vi "oa_Multichannel dr Check.vi"(8 "error in (no error)":errorcluster, 11 "resampled signal in":cluster{"r0":dbl, "dr":dbl, "Y":dbl[]}[](array[cluster]) {"r0" format="%.2p"; "dr" format="%.2p"; "Y" format="%.2f"}) -> (0 "error out":errorcluster, 2 "empty signal":bool, 3 "resampled signal out":cluster{"r0":dbl, "dr":dbl, "Y":dbl[]}[](array[cluster]))   [LabVIEW 2017, in "SoundVib_Resampling.lvlib"]
uses:
  <vilib>/addons/Sound and Vibration/Order Analysis/Resample Order Tracking/SoundVib_Resampling.lvlib
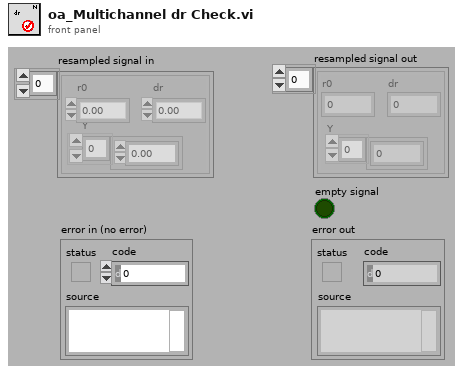
[diagram p1: front panel]
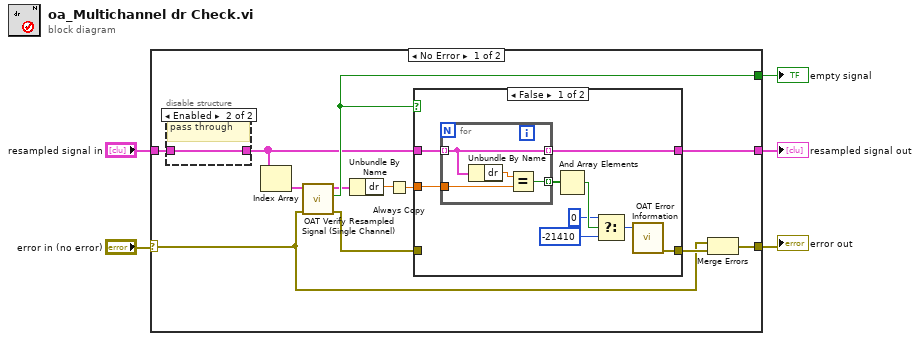
[diagram p0: block diagram]
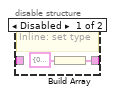
[diagram p2: hidden frame]
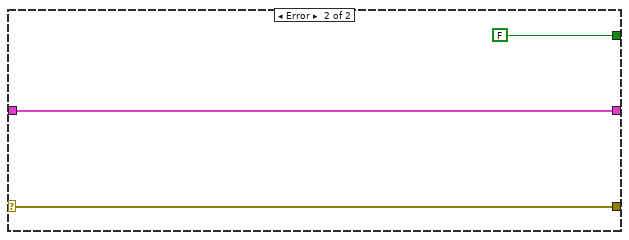
[diagram p4: hidden frame]
diagram:
  n1 = case shown="No Error" "error in (no error)" {
    selector: "error in (no error)" -> [w12 w37]
    tunnel: [w17 w38] -> w5
    tunnel: "resampled signal in" -> [w6 w38]
    tunnel: [w16 w37] -> w2
    tunnel: [w13 FALSE] -> w1
    frame No Error {
      n2 = disable-structure shown="Enabled" {
        disable-tunnel: [w18 w20] -> w7
        disable-tunnel: w6 -> [_ w20]
        frame Disabled {
          # "Inline: set type"
          n3 = Build Array(cluster{"r0":dbl, "dr":dbl, "Y":dbl[]} {"r0"=0.0, "dr"=0.0, "Y"=[]} ("resampled signal")) -> (w18:cluster{"r0":dbl, "dr":dbl, "Y":dbl[]}[])
        }
        frame Enabled {
          # "pass through"
        }
      }
      n4 = Index Array(array=w7) -> (element=w14:cluster{"r0":dbl, "dr":dbl, "Y":dbl[]})  [unwired: 1 in]
      n5 = call <vilib>:"OAT Verify Resampled Signal (Single Channel).vi"("error in (no error)"=w12, "resampled signal"=w14) -> ("error out"=w11:errorcluster, "empty signal?"=w13:bool, "resampled signal dup"=w10:cluster{"r0":dbl, "dr":dbl, "Y":dbl[]})  [unwired: 7 in]
      n6 = Unbundle By Name(w10) -> ("dr"=w9:dbl)
      n7 = Always Copy(1:w9) -> (0:w8:dbl)
      n8 = case shown="False" w13 {
        tunnel: [w29 w35] -> w17
        tunnel: w7 -> [w24 w35]
        tunnel: [w22 w34] -> w15
        tunnel: w11 -> [_ w34]
        tunnel: w8 -> [w21 _]
        frame False {
          n9 = for {
            tunnel: w24 -> [w33] mode=indexing
            tunnel: [w33] -> w29 mode=indexing
            tunnel: w21 -> [w32]
            tunnel: [w30] -> w28 mode=indexing
            n10 = Unbundle By Name(w33) -> ("dr"=w31:dbl)
            n11 = Equal?(x=w31, y=w32) -> (x = y?=w30:bool)
          }
          n12 = And Array Elements(Boolean array=w28) -> (logical AND=w27:bool)
          n13 = Select(t=0, s=w27, f=-21410) -> (s? t:f=w23:i32)
          n14 = call <vilib>:"OAT Error Information.vi"("error code"=w23) -> ("error out"=w22:errorcluster)  [unwired: 6 in]
        }
        frame True {
        }
      }
      n15 = Merge Errors(w12, w15) -> (w16:errorcluster)
    }
    frame Error {
    }
  }
  "resampled signal out" <- w5
  "error out" <- w2
  "empty signal" <- w1
